vi "Print.vi"(8 "Error In":errorcluster, 11 "reference in":refnum<class "MenuItem.lvclass">) -> (0 "Error Out":errorcluster, 3 "reference in":refnum<class "MenuItem.lvclass">)   [LabVIEW 2020, in "MenuItem.lvclass"]
uses:
  MenuItem.lvclass
  Console_class/Console.lvclass
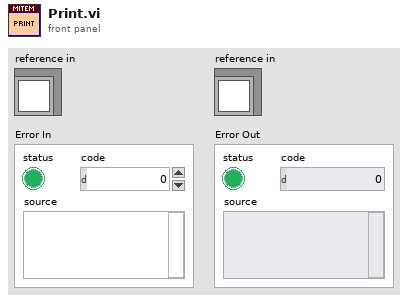
[diagram p1: front panel]
types:
  T1 = typedef "MenuItem.lvclass/ObjectAttributes.ctl" = cluster{"Name":string, "Description":string, "Price":dbl, "Vegetarian":bool}
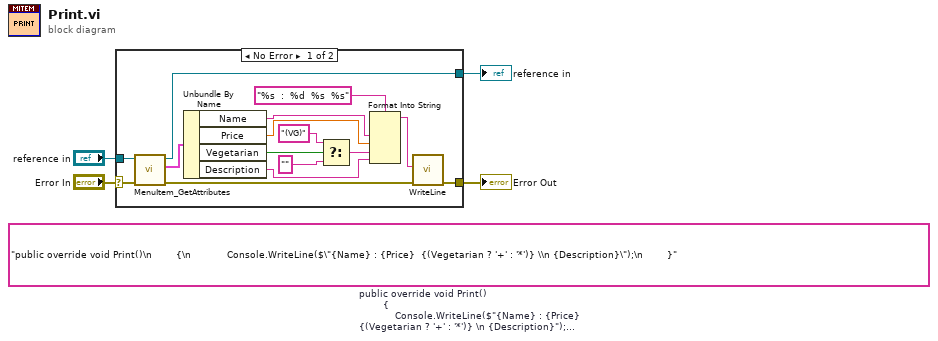
[diagram p0: block diagram]
diagram:
  (unwired) "public override void Print()\n        {\n            Console.WriteLine($\"{Name} : {Price}  {(Vegetarian ? '+' : '*')} \\n {Description}\");\n        }"  # public override void Print()         {             Console.WriteLine($"{Name} : {Price}  {(Vegetarian ? '+' : '*')} \n {Description}");         }
  n1 = case shown="No Error" "Error In" {
    selector: "Error In" -> [w18 w21]
    tunnel: [w6 w21] -> w3
    tunnel: [w17 w20] -> w1
    tunnel: "reference in" -> [w19 w20]
    frame No Error {
      n2 = call "MenuItem_GetAttributes.vi"("error in (no error)"=w18, "reference in"=w19) -> ("error out"=w7:errorcluster, "Data"=w8:T1, "reference out"=w17:refnum<class "MenuItem.lvclass">)  [unwired: 6 in, 1 out]
      n3 = Unbundle By Name(w8) -> ("Name"=w16:string, "Price"=w15:dbl, "Vegetarian"=w13:bool, "Description"=w14:string)
      n4 = Select(t="(VG)", s=w13, f="") -> (s? t:f=w5:string)
      n5 = Format Into String(format string="%s  :  %d  %s  %s", w16, w15, w5, w14) -> (resulting string=w9:string)  [unwired: 2 in, 1 out]
      n6 = call "WriteLine.vi"("Error In"=w7, "ConsoleText"=w9) -> ("Error Out"=w6:errorcluster)  [unwired: 9 in]
    }
    frame Error {
    }
  }
  "Error Out" <- w3
  "reference in" <- w1
